vi "ma_SML Spectrum.vi"   [LabVIEW 2020, in "NI_MAPro.lvlib"]
uses:
  NI_MAPro.lvlib
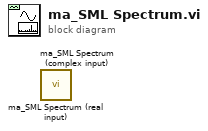
[diagram p0: block diagram]
diagram:
  n1 = call "ma_SML Spectrum (real input).vi"() -> ()  [unwired: 3 in, 2 out]
  n2 = call "ma_SML Spectrum (complex input).vi"() -> ()  [unwired: 3 in, 2 out]
